vi "LDA_span_and_centre.vi"(2 "Calibration factor":dbl=3.97 format="%.4f", 3 "Frequency shift":enum16{"Disabled", "Enabled"}(ring)=enum."Enabled", 4 "Units":enum16{"Hz", "m/s"}(ring)=enum."m/s", 5 "Velocity span":u16=10) -> (0 "Centres":dbl[](array[numeric]), 1 "Spans":dbl[](array[numeric]))   [LabVIEW 2010]
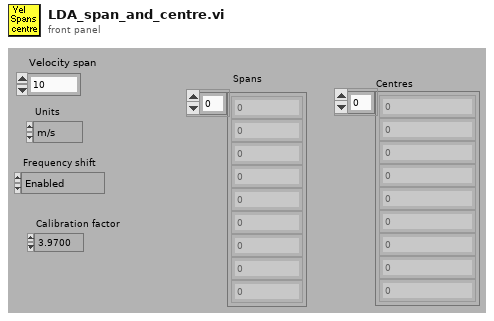
[diagram p1: front panel]
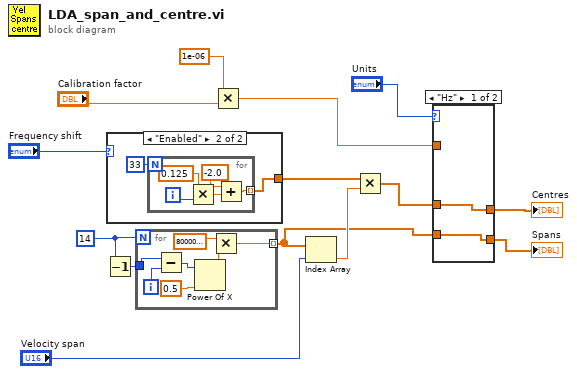
[diagram p0: block diagram]
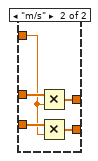
[diagram p2: hidden frame]
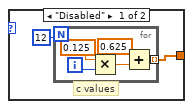
[diagram p3: hidden frame]
diagram:
  w11 = 14
  n1 = Decrement(x=w11) -> (x-1=w12:i32)
  n2 = case shown="\"Enabled\"" "Frequency shift" {
    tunnel: [w15 w22] -> w14
    frame "Disabled" {
      # "c values"
      n3 = for {
        N: 12 -> [_]
        tunnel: [w17] -> w15 mode=indexing
        i -> [w18]
        n4 = Multiply(x=0.125, y=w18) -> (x*y=w20:dbl)
        n5 = Add(x=0.625, y=w20) -> (x+y=w17:dbl)
      }
    }
    frame "Enabled" {
      n6 = for {
        N: 33 -> [_]
        tunnel: [w24] -> w22 mode=indexing
        i -> [w25]
        n7 = Multiply(x=0.125, y=w25) -> (x*y=w27:dbl)
        n8 = Add(x=-2.0, y=w27) -> (x+y=w24:dbl)
      }
    }
  }
  n9 = for {
    N: w11 -> [_]
    tunnel: w12 -> [w30]
    tunnel: [w29] -> w8 mode=indexing
    i -> [w35]
    n10 = Subtract(x=w30, y=w35) -> (x-y=w33:i32)
    n11 = Power Of X(1:0.5, 2:w33) -> (0:w32:dbl)
    n12 = Multiply(x=8000000.0, y=w32) -> (x*y=w29:dbl)
  }
  n13 = Multiply(x=1e-06, y="Calibration factor") -> (x*y=w9:dbl)
  n14 = Index Array(array=w8, index="Velocity span") -> (element=w13:dbl)
  n15 = Multiply(x=w14, y=w13) -> (x*y=w7:dbl[])
  n16 = case shown="\"Hz\"" "Units" {
    tunnel: w9 -> [_ w38]
    tunnel: w7 -> [w37 w42]
    tunnel: w8 -> [w36 w41]
    tunnel: [w37 w40] -> w6
    tunnel: [w36 w39] -> w5
    frame "Hz" {
    }
    frame "m/s" {
      n17 = Multiply(x=w42, y=w38) -> (x*y=w40:dbl[])
      n18 = Multiply(x=w41, y=w38) -> (x*y=w39:dbl[])
    }
  }
  "Centres" <- w6
  "Spans" <- w5
